vi "module disconnect And Destory Stem.vi"(7 "dll path in":path, 8 "error in (no error)":errorcluster, 10 "result":cluster{"value":i32, "error":i32}, 11 "id":u32) -> (0 "error out":errorcluster, 2 "result out":cluster{"value":i32, "error":i32}, 3 "id out":u32)   [LabVIEW 2025]
doc: "aLIBEXPORT void __stdcall module_disconnectAndDestoryStem(unsigned int* id, struct Result* result);"
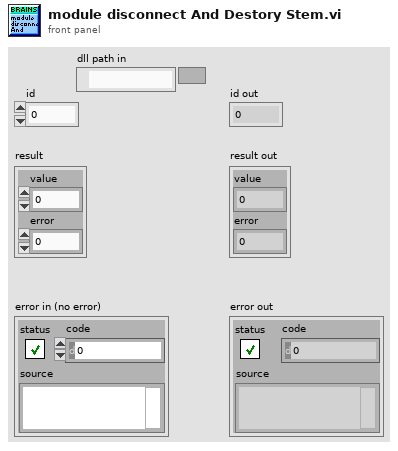
[diagram p1: front panel]
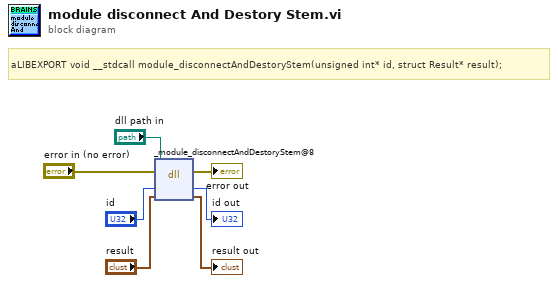
[diagram p0: block diagram]
diagram:
  # "aLIBEXPORT void __stdcall module_disconnectAndDestoryStem(unsigned int* id, struct Result* result);"
  n1 = dll-call lib="?" fn="_module_disconnectAndDestoryStem@8"(path in="dll path in", error in="error in (no error)", "id"="id", "result"="result") -> (error out=→"error out":errorcluster, "id"=→"id out":u32, "result"=→"result out":cluster{"value":i32, "error":i32})  [unwired: 2 in, 1 out]
